vi "Teleop.vi"(10 "Match Info":T1={"Autonomous Elapsed Seconds"=0.0, "TeleOp Elapsed Seconds"=0.0, "Disabled Elapsed Seconds"=0.0, "Visited Autonomous"=FALSE, "Visited TeleOp"=FALSE, "Visited Disabled"=FALSE, "Autonomous Settings"={"Autonomous Style"=enum."Independent", "VI Refnum"=refnum}}, 11 "Call Context":T2) -> ()   [LabVIEW 2019]
doc: "This VI is called for each TeleOp packet received from the DS where the robot is not disabled. It is often used to read from the joysticks and update I/O or to update setpoints for timed control loops. It should complete and return within 20 milliseconds or it may miss DS packets."
uses:
  <vilib>/Rock Robotics/Network Tables/NT Write Boolean Array.vi
  <vilib>/Rock Robotics/Network Tables/NT Read Boolean.vi
  2019 Robot Project/Joystick_Buttons.vi
  2019 Robot Project/GlobalRefnum.vi
  <vilib>/Rock Robotics/WPI/ThirdParty/Phoenix-LabVIEW/Motor Controller/Controls/CTRE_Phoenix_MotorControl_ControlMode.ctl
  <vilib>/Rock Robotics/Network Tables/NT Read Number.vi
  <vilib>/Rock Robotics/WPI/DriverStation/WPI_DriverStationMatch Info.ctl
  <vilib>/Rock Robotics/WPI/DriverStation/WPI_DriverStationDerivedRobotMode.ctl
panel:
  out "Sample Slider 0":dbl(slide) scale=0.0..5.0
  out "Sample Boolean 1":bool
  out "Sample Boolean 0":bool
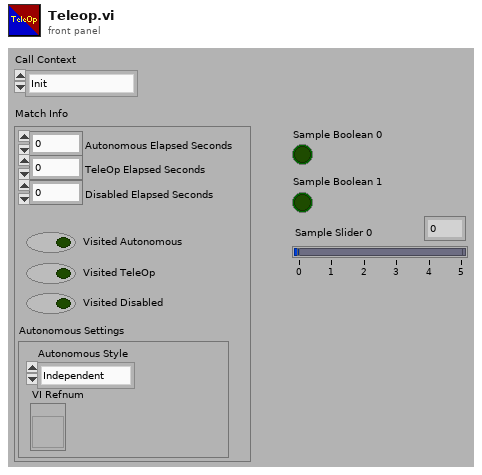
[diagram p1: front panel]
types:
  T1 = typedef "WPI_DriverStationMatch Info.ctl" = cluster{"Autonomous Elapsed Seconds":dbl, "TeleOp Elapsed Seconds":dbl, "Disabled Elapsed Seconds":dbl, "Visited Autonomous":bool, "Visited TeleOp":bool, "Visited Disabled":bool, "Autonomous Settings":cluster{"Autonomous Style":enum16{"Iterative", "Independent"}, "VI Refnum":refnum<vi>}}
  T2 = typedef "WPI_DriverStationDerivedRobotMode.ctl" = enum16{"Init", "Execute", "Stop"}
  T3 = typedef "CTRE_Phoenix_MotorControl_ControlMode.ctl" = u16
  T4 = typedef "WPI_JoystickDevRef.ctl" = cluster{"Device":T5}
  T5 = typedef "WPI_JoystickDeviceEnum.ctl" = enum16{"USB 0", "USB 1", "USB 2", "USB 3", "USB 4", "USB 5"}
  T6 = cluster{"Axes[0]":dbl, "Axes[1]":dbl, "Axes[2]":dbl, "Axes[3]":dbl, "Axes[4]":dbl, "Axes[5]":dbl, "Axes[6]":dbl, "Axes[7]":dbl, "Axes[8]":dbl}
  T7 = cluster{"Buttons[0]":bool, "Buttons[1]":bool, "Buttons[2]":bool, "Buttons[3]":bool, "Buttons[4]":bool, "Buttons[5]":bool, "Buttons[6]":bool, "Buttons[7]":bool, "Buttons[8]":bool}
  T8 = typedef "WPI_MotorControlDeviceRef.ctl" = cluster{"DeviceStatus":errorcluster, "Type":T9, "PWM":cluster{"PWM Channel":T10, "DeadBand":T11}, "CAN":cluster{"Device Number":u8, "SetOutput VI Ref":variant, "GetOutput VI Ref":variant, "Enable VI Ref":variant, "Disable VI Ref":variant, "Data":variant}, "Invert":bool, "DIO PWM":cluster{"PWM \"Enable\" Channel":T10, "DIOChannel":T12, "PWM Rate":dbl}}
  T9 = typedef "WPI_MotorControlType.ctl" = enum16{"PWM", "CAN", "DIO PWM"}
  T10 = typedef "FPGA_DIOPWMChannel.ctl" = enum8{"PWM 0", "PWM 1", "PWM 2", "PWM 3", "PWM 4", "PWM 5", "PWM 6", "PWM 7", "PWM 8", "PWM 9", "PWM MXP 0", "PWM MXP 1", "PWM MXP 2", "PWM MXP 3", "PWM MXP 4", "PWM MXP 5", "PWM MXP 6", "PWM MXP 7", "PWM MXP 8", "PWM MXP 9", "Invalid"}
  T11 = typedef "WPI_PWMDeadband.ctl" = cluster{"Name":string, "maxPositivePwm":i32, "minPositivePwm":i32, "centerPwm":i32, "maxNegativePwm":i32, "minNegativePwm":i32, "angularRange":u16}
  T12 = typedef "FPGA_DIOChannel.ctl" = enum8{"DIO 0", "DIO 1", "DIO 2", "DIO 3", "DIO 4", "DIO 5", "DIO 6", "DIO 7", "DIO 8", "DIO 9", "DIO MXP 0", "DIO MXP 1", "DIO MXP 2", "DIO MXP 3", "DIO MXP 4", "DIO MXP 5", "DIO MXP 6", "DIO MXP 7", "DIO MXP 8", "DIO MXP 9", "DIO MXP 10", "DIO MXP 11", "DIO MXP 12", "DIO MXP 13", "DIO MXP 14", "DIO MXP 15", "SPI Port CS1", "SPI Port CS2", "SPI Port CS3", "SPI Port MISO", "SPI Port MOSI", "Invalid"}
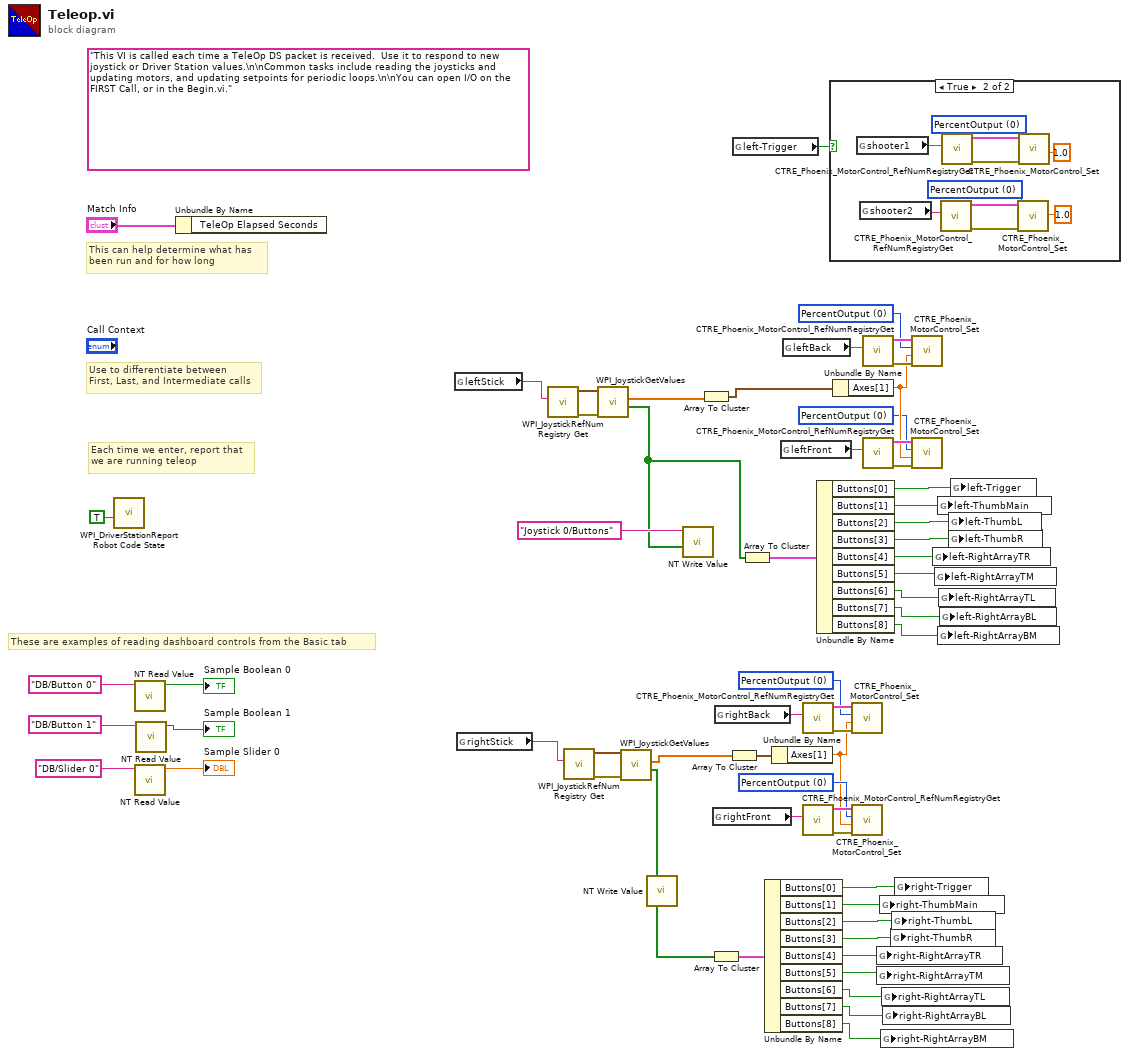
[diagram p0: block diagram]
diagram:
  w6 = T3 0 items=["PercentOutput"=0, "Position"=1, "Velocity"=2, "Current"=3, "Follower"=5, "MotionProfile"=6, "MotionMagic"=7, "MotionProfileArc"=10, "Disabled"=15] ("Control Mode")
  w10 = T3 0 items=["PercentOutput"=0, "Position"=1, "Velocity"=2, "Current"=3, "Follower"=5, "MotionProfile"=6, "MotionMagic"=7, "MotionProfileArc"=10, "Disabled"=15] ("Control Mode")
  w30 = T3 0 items=["PercentOutput"=0, "Position"=1, "Velocity"=2, "Current"=3, "Follower"=5, "MotionProfile"=6, "MotionMagic"=7, "MotionProfileArc"=10, "Disabled"=15] ("Control Mode")
  w31 = T3 0 items=["PercentOutput"=0, "Position"=1, "Velocity"=2, "Current"=3, "Follower"=5, "MotionProfile"=6, "MotionMagic"=7, "MotionProfileArc"=10, "Disabled"=15] ("Control Mode")
  (unwired) "This VI is called each time a TeleOp DS packet is received.  Use it to respond to new joystick or Driver Station values.\n\nCommon tasks include reading the joysticks and updating motors, and updating setpoints for periodic loops.\n\nYou can open I/O on the FIRST Call, or in the Begin.vi."
  # "These are examples of reading dashboard controls from the Basic tab"
  # "Each time we enter, report that\nwe are running teleop"
  # "Use to differentiate between\nFirst, Last, and Intermediate calls"
  # "This can help determine what has\nbeen run and for how long"
  n1 = call <vilib>:"WPI_DriverStationReport Robot Code State.vi"("TeleOp"=TRUE ("Autonomous")) -> ()  [unwired: 10 in, 1 out]
  n2 = call-poly <vilib>:"NT Read Value.vi"("Name"="DB/Button 0" ("refnum name")) -> ("Boolean"=→"Sample Boolean 0":bool)  [unwired: 9 in, 1 out]
  n3 = call-poly <vilib>:"NT Read Value.vi"("Name"="DB/Slider 0" ("refnum name")) -> ("Numeric"=→"Sample Slider 0":dbl)  [unwired: 9 in, 1 out]
  n4 = call-poly <vilib>:"NT Read Value.vi"("Name"="DB/Button 1" ("refnum name")) -> ("Boolean"=→"Sample Boolean 1":bool)  [unwired: 9 in, 1 out]
  n5 = Unbundle By Name("Match Info") -> ()  [unwired: 1 out]
  n6 = global read "GlobalRefnum.vi" "leftStick"() -> (w41:string)
  n7 = global read "GlobalRefnum.vi" "rightStick"() -> (w14:string)
  n8 = call <vilib>:"WPI_JoystickRefNum Registry Get.vi"("refnum name"=w41) -> ("error out"=w27:errorcluster, "JoystickDevRef"=w59:T4)  [unwired: 1 in, 8 out]
  n9 = call <vilib>:"WPI_JoystickRefNum Registry Get.vi"("refnum name"=w14) -> ("error out"=w28:errorcluster, "JoystickDevRef"=w29:T4)  [unwired: 9 in]
  n10 = call <vilib>:"WPI_JoystickGetValues.vi"("error in (no error)"=w27, "JoystickDevRef"=w59) -> ("Buttons"=w2:bool[], "Axes"=w40:dbl[])  [unwired: 5 in, 3 out]
  n11 = call <vilib>:"WPI_JoystickGetValues.vi"("error in (no error)"=w28, "JoystickDevRef"=w29) -> ("Buttons"=w15:bool[], "Axes"=w26:dbl[])  [unwired: 5 in, 3 out]
  n12 = call-poly <vilib>:"NT Write Value.vi"("Boolean Array"=w15) -> ()  [unwired: 10 in, 1 out]
  n13 = call-poly <vilib>:"NT Write Value.vi"("Boolean Array"=w2, "Name"="Joystick 0/Buttons") -> ()  [unwired: 9 in, 1 out]
  n14 = Array To Cluster(array=w40) -> (cluster=w39:T6)
  n15 = Array To Cluster(array=w15) -> (cluster=w4:T7)
  n16 = global read "GlobalRefnum.vi" "rightFront"() -> (w7:string)
  n17 = global read "GlobalRefnum.vi" "rightBack"() -> (w11:string)
  n18 = Array To Cluster(array=w26) -> (cluster=w25:T6)
  n19 = global read "Joystick_Buttons.vi" "left-Trigger"() -> (w1:bool)
  n20 = Array To Cluster(array=w2) -> (cluster=w3:T7)
  n21 = Unbundle By Name(w4) -> ("Buttons[0]"=w24:bool, "Buttons[1]"=w23:bool, "Buttons[2]"=w22:bool, "Buttons[3]"=w21:bool, "Buttons[4]"=w20:bool, "Buttons[5]"=w19:bool, "Buttons[6]"=w18:bool, "Buttons[7]"=w17:bool, "Buttons[8]"=w16:bool)
  n22 = Unbundle By Name(w25) -> ("Axes[1]"=w5:dbl)
  n23 = global read "GlobalRefnum.vi" "leftFront"() -> (w34:string)
  n24 = global read "GlobalRefnum.vi" "leftBack"() -> (w33:string)
  n25 = call <vilib>:"CTRE_Phoenix_MotorControl_RefNumRegistryGet.vi"("refnum name"=w11) -> ("error out"=w13:errorcluster, "PhoenixMotorControlDevRef"=w12:T8)  [unwired: 9 in]
  n26 = call <vilib>:"CTRE_Phoenix_MotorControl_RefNumRegistryGet.vi"("refnum name"=w7) -> ("error out"=w9:errorcluster, "PhoenixMotorControlDevRef"=w8:T8)  [unwired: 9 in]
  n27 = Unbundle By Name(w3) -> ("Buttons[0]"=w50:bool, "Buttons[1]"=w49:bool, "Buttons[2]"=w48:bool, "Buttons[3]"=w47:bool, "Buttons[4]"=w46:bool, "Buttons[5]"=w45:bool, "Buttons[6]"=w44:bool, "Buttons[7]"=w43:bool, "Buttons[8]"=w42:bool)
  n28 = case shown="True" w1 {
    frame False {
    }
    frame True {
      w63 = T3 0 items=["PercentOutput"=0, "Position"=1, "Velocity"=2, "Current"=3, "Follower"=5, "MotionProfile"=6, "MotionMagic"=7, "MotionProfileArc"=10, "Disabled"=15] ("Control Mode")
      w64 = T3 0 items=["PercentOutput"=0, "Position"=1, "Velocity"=2, "Current"=3, "Follower"=5, "MotionProfile"=6, "MotionMagic"=7, "MotionProfileArc"=10, "Disabled"=15] ("Control Mode")
      n29 = global read "GlobalRefnum.vi" "shooter1"() -> (w62:string)
      n30 = global read "GlobalRefnum.vi" "shooter2"() -> (w61:string)
      n31 = call <vilib>:"CTRE_Phoenix_MotorControl_RefNumRegistryGet.vi"("refnum name"=w61) -> ("error out"=w67:errorcluster, "PhoenixMotorControlDevRef"=w68:T8)  [unwired: 9 in]
      n32 = call <vilib>:"CTRE_Phoenix_MotorControl_RefNumRegistryGet.vi"("refnum name"=w62) -> ("error out"=w69:errorcluster, "PhoenixMotorControlDevRef"=w70:T8)  [unwired: 9 in]
      n33 = call <vilib>:"CTRE_Phoenix_MotorControl_Set.vi"("error in (no error)"=w67, "Output"=1.0, "Control Mode"=w64, "PhoenixMotorControlDevRef"=w68) -> ()  [unwired: 6 in, 2 out]
      n34 = call <vilib>:"CTRE_Phoenix_MotorControl_Set.vi"("error in (no error)"=w69, "Output"=1.0, "Control Mode"=w63, "PhoenixMotorControlDevRef"=w70) -> ()  [unwired: 6 in, 2 out]
    }
  }
  n35 = Unbundle By Name(w39) -> ("Axes[1]"=w32:dbl)
  n36 = call <vilib>:"CTRE_Phoenix_MotorControl_Set.vi"("error in (no error)"=w13, "Output"=w5, "Control Mode"=w10, "PhoenixMotorControlDevRef"=w12) -> ()  [unwired: 6 in, 2 out]
  n37 = call <vilib>:"CTRE_Phoenix_MotorControl_Set.vi"("error in (no error)"=w9, "Output"=w5, "Control Mode"=w6, "PhoenixMotorControlDevRef"=w8) -> ()  [unwired: 6 in, 2 out]
  n38 = call <vilib>:"CTRE_Phoenix_MotorControl_RefNumRegistryGet.vi"("refnum name"=w33) -> ("error out"=w36:errorcluster, "PhoenixMotorControlDevRef"=w35:T8)  [unwired: 9 in]
  n39 = call <vilib>:"CTRE_Phoenix_MotorControl_RefNumRegistryGet.vi"("refnum name"=w34) -> ("error out"=w37:errorcluster, "PhoenixMotorControlDevRef"=w38:T8)  [unwired: 9 in]
  n40 = global write "Joystick_Buttons.vi" "right-RightArrayTR"(w20) -> ()
  n41 = global write "Joystick_Buttons.vi" "right-RightArrayTM"(w19) -> ()
  n42 = global write "Joystick_Buttons.vi" "right-ThumbMain"(w23) -> ()
  n43 = global write "Joystick_Buttons.vi" "right-RightArrayBM"(w16) -> ()
  n44 = global write "Joystick_Buttons.vi" "right-RightArrayTL"(w18) -> ()
  n45 = global write "Joystick_Buttons.vi" "right-RightArrayBL"(w17) -> ()
  n46 = global write "Joystick_Buttons.vi" "right-ThumbR"(w21) -> ()
  n47 = global write "Joystick_Buttons.vi" "right-ThumbL"(w22) -> ()
  n48 = global write "Joystick_Buttons.vi" "right-Trigger"(w24) -> ()
  n49 = call <vilib>:"CTRE_Phoenix_MotorControl_Set.vi"("error in (no error)"=w36, "Output"=w32, "Control Mode"=w31, "PhoenixMotorControlDevRef"=w35) -> ()  [unwired: 6 in, 2 out]
  n50 = call <vilib>:"CTRE_Phoenix_MotorControl_Set.vi"("error in (no error)"=w37, "Output"=w32, "Control Mode"=w30, "PhoenixMotorControlDevRef"=w38) -> ()  [unwired: 6 in, 2 out]
  n51 = global write "Joystick_Buttons.vi" "left-RightArrayTR"(w46) -> ()
  n52 = global write "Joystick_Buttons.vi" "left-RightArrayTM"(w45) -> ()
  n53 = global write "Joystick_Buttons.vi" "left-ThumbMain"(w49) -> ()
  n54 = global write "Joystick_Buttons.vi" "left-RightArrayBM"(w42) -> ()
  n55 = global write "Joystick_Buttons.vi" "left-RightArrayTL"(w44) -> ()
  n56 = global write "Joystick_Buttons.vi" "left-RightArrayBL"(w43) -> ()
  n57 = global write "Joystick_Buttons.vi" "left-ThumbL"(w48) -> ()
  n58 = global write "Joystick_Buttons.vi" "left-ThumbR"(w47) -> ()
  n59 = global write "Joystick_Buttons.vi" "left-Trigger"(w50) -> ()
